vi "Get Scanner.vi"(8 "error in (no error)":errorcluster, 11 "Lakeshore Gaussmeter in":refnum<class "Lakeshore Gaussmeter.lvclass">) -> (0 "error out":errorcluster, 2 "Default Scanner out":refnum<class "Scanner.lvclass">)   [LabVIEW 2017, in "Lakeshore Gaussmeter.lvclass"]
doc: "(Dynamic) Returns the default Scanner object that scans over this Scannable. (Note that a Scannable may have multiple Scanners associated with it.) A Scanner is an analogue to an Iterator class in other languages."
uses:
  Lakeshore Gaussmeter.lvclass
  Scanners/Scanner/Scanner.lvclass
  Scanners/Magnetic Field Lakeshore/Magnetic Field Lakeshore Scan.lvclass
  C:/LabVIEW-programs/Scanners/Scanner/Scanner.lvclass
  Utility Classes/Scannable/Scannable.lvclass
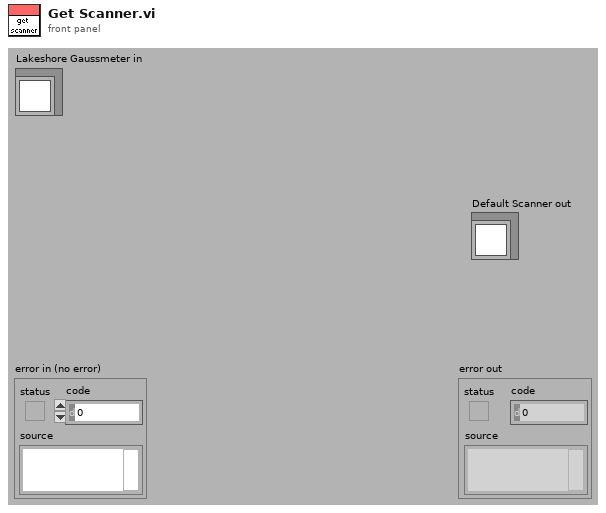
[diagram p1: front panel]
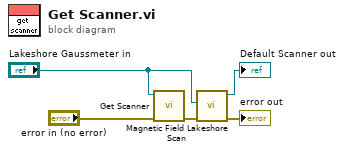
[diagram p0: block diagram]
diagram:
  n1 = call-parent "Get Scanner.vi"("error in (no error)"="error in (no error)", "Scannable in"="Lakeshore Gaussmeter in") -> ("error out"=w2:errorcluster)  [unwired: 8 in, 1 out]
  n2 = call "Magnetic Field Lakeshore Scan.vi"("error in (no error)"=w2, "Lakeshore Gaussmeter.lvclass"="Lakeshore Gaussmeter in") -> ("error out"=→"error out":errorcluster, "Magnetic Field Lakeshore Scan out"=→"Default Scanner out":refnum<class "Magnetic Field Lakeshore Scan.lvclass">)  [unwired: 8 in]
